vi "Lock_LO_RevB_digitalPLL_NAOJ_2.vi"(0 "ObjHandle in":u32, 2 "LO_FREQ_SET":T1={"YTO Low freq. [GHz]"=12.17, "YTO High freq. [GHz]"=14.833, "Kvco"=1, "Lock Pol."=0, "SET LO FREQ"=25.0, "Multiplier"=3.0, "YTO coarse tune(HEX)"=0, "YTO coarse( FREQ)"=25.0, "NULL PLL INTEGRATOR"=FALSE} {"YTO coarse( FREQ)" min=25 max=150 step=0.0001 format="%.3f"; "YTO coarse tune(HEX)" format="%x"; "Multiplier" min=3 max=6 step=3; "SET LO FREQ" min=25 max=150 step=0.0001 format="%.3f"; "Lock Pol." items=["Lower", "Upper"]; "Kvco" items=["7.5MHz/V", "15MHz/V"]; "YTO High freq. [GHz]" format="%.3f"; "YTO Low freq. [GHz]" format="%.3f"}, 5 "error in (no error)":errorcluster, 10 "Slave Node in":cluster{"Address":i16, "Serial Number":i8[]}={"Address"=19, "Serial Number"=[16, 71, 55, 76, 1, 8, 0, -15]} {"Serial Number" format="%.0x"; "Address" format="%.0x"}, 12 "Cartridge band":u32 max=10 step=1) -> (15 "LO_FREQ_output":T1={"YTO Low freq. [GHz]"=12.17, "YTO High freq. [GHz]"=14.833, "Kvco"=1, "Lock Pol."=0, "SET LO FREQ"=25.0, "Multiplier"=3.0, "YTO coarse tune(HEX)"=0, "YTO coarse( FREQ)"=25.0, "NULL PLL INTEGRATOR"=FALSE} {"YTO coarse( FREQ)" min=25 max=150 step=0.0001 format="%.3f"; "YTO coarse tune(HEX)" format="%x"; "Multiplier" min=3 max=6 step=3; "SET LO FREQ" min=25 max=150 step=0.0001 format="%.3f"; "Lock Pol." items=["Lower", "Upper"]; "Kvco" items=["7.5MHz/V", "15MHz/V"]; "YTO High freq. [GHz]" format="%.3f"; "YTO Low freq. [GHz]" format="%.3f"}, 16 "YTO final Freq [GHz]":sgl format="%.4f", 17 "YTO fine  Freq [GHz]":sgl format="%.4f", 19 "error out":errorcluster)   [LabVIEW 2017]
panel:
  in  "step(GHz)":sgl=0.001
  out "l":dbl
  out "ObjHandle out":u32
  # "LO freq. [GHz]"
  # "ZERO Intgrtr"
  # "LO freq. [GHz]"
  # "ZERO Intgrtr"
  # "Node Address"
  # "Serial Number"
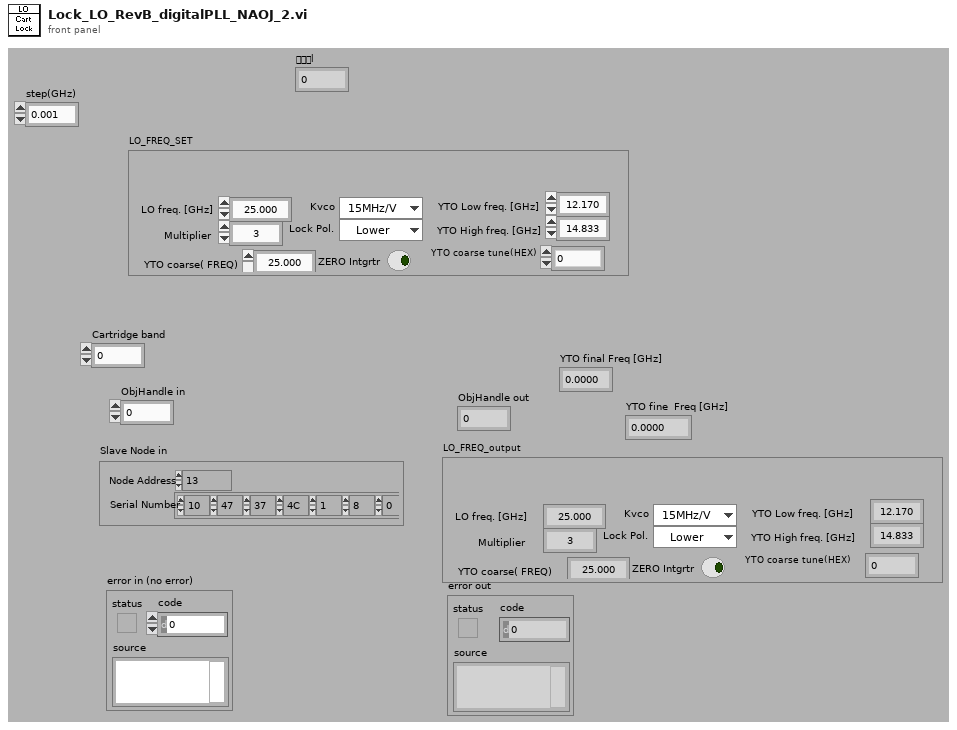
[diagram p1: front panel]
types:
  T1 = cluster{"YTO Low freq. [GHz]":sgl, "YTO High freq. [GHz]":sgl, "Kvco":u16, "Lock Pol.":u16, "SET LO FREQ":sgl, "Multiplier":sgl, "YTO coarse tune(HEX)":u16, "YTO coarse( FREQ)":sgl, "NULL PLL INTEGRATOR":bool}
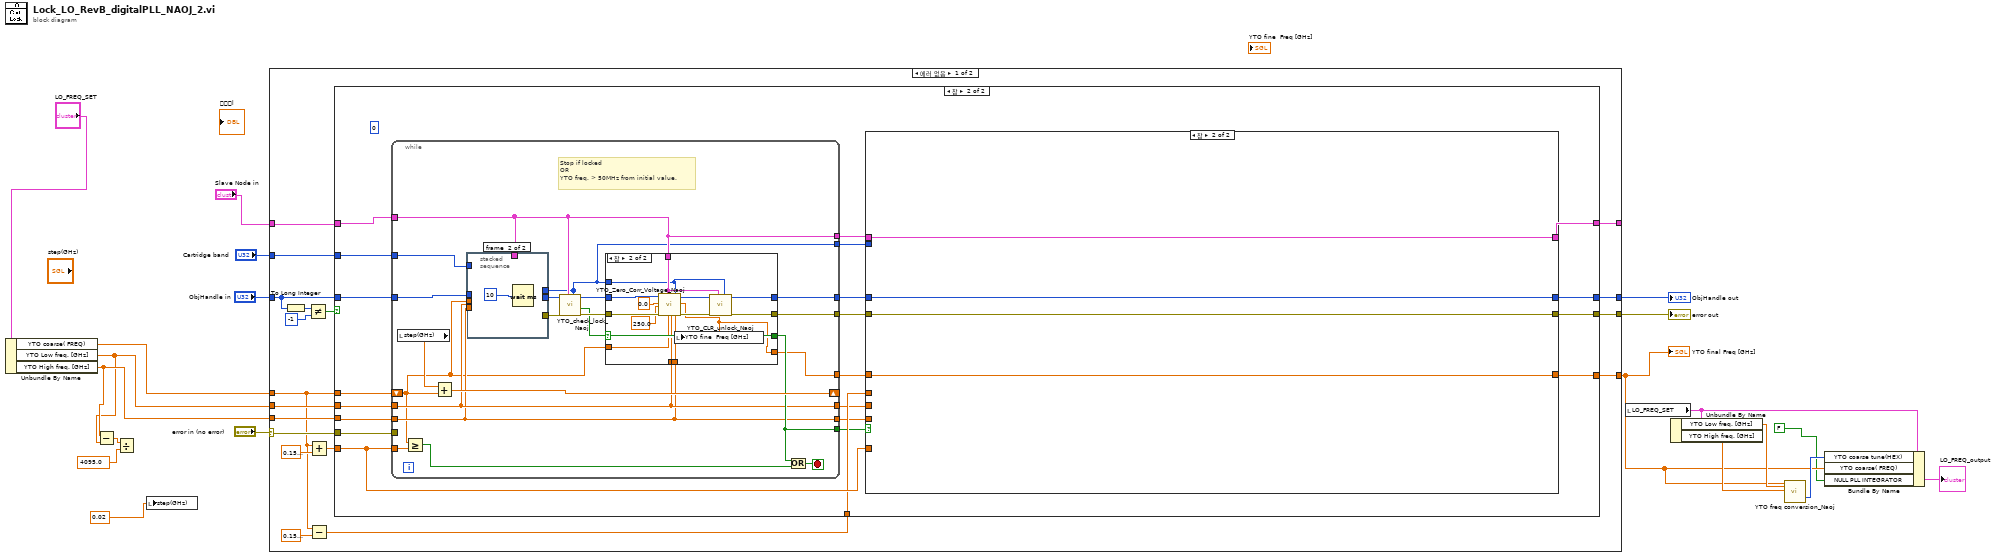
[diagram p0: block diagram]
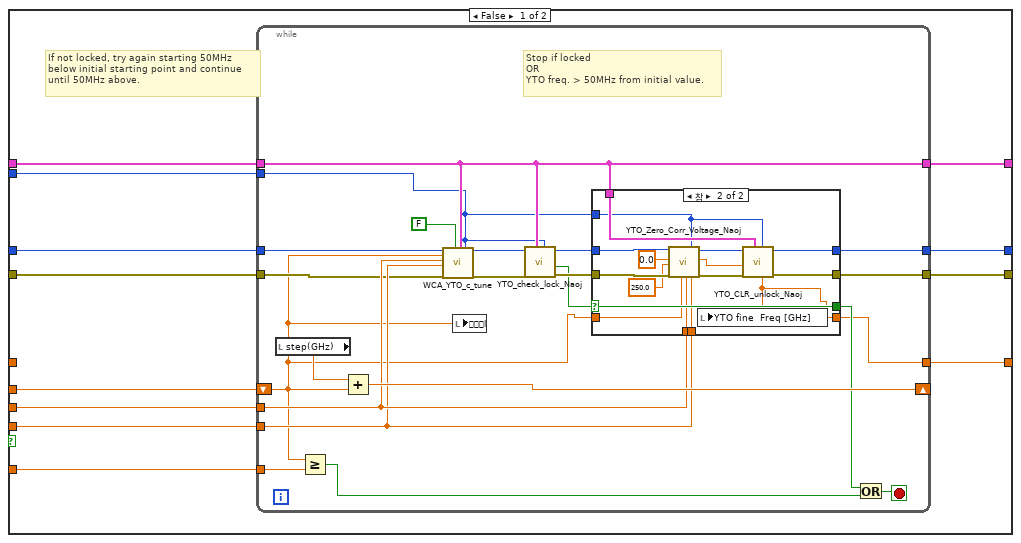
[diagram p3: hidden frame]
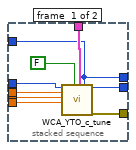
[diagram p5: hidden frame]
diagram:
  n1 = Unbundle By Name("LO_FREQ_SET") -> ("YTO coarse( FREQ)"=w13:sgl, "YTO Low freq. [GHz]"=w2:sgl, "YTO High freq. [GHz]"=w3:sgl)
  n2 = Subtract(x=w3, y=w2) -> (x-y=w5:sgl)
  n3 = Divide(x=w5, y=4095.0) -> ()  [unwired: 1 out]
  n4 = local write "step(GHz)"(0.02) -> ()
  n5 = case shown="에러 없음" "error in (no error)" {
    selector: "error in (no error)" -> [w35 w174]
    tunnel: "ObjHandle in" -> [w34 w172]
    tunnel: "Slave Node in" -> [w33 w173]
    tunnel: w2 -> [w32 _]
    tunnel: w3 -> [w31 _]
    tunnel: w13 -> [w23 _]
    tunnel: [w30 w172] -> w17
    tunnel: [w29 w173] -> _
    tunnel: [w28 w174] -> w18
    tunnel: [w25 sgl -1.0 ("SET YTO COARSE TUNE")] -> w7
    tunnel: "Cartridge band" -> [w21 _]
    frame No Error {
      n6 = To Long Integer(number=w34) -> (32bit integer=w37:i32)
      n7 = Not Equal?(x=w37, y=-1) -> (x != y?=w36:bool)
      n8 = Add(x=w23, y=sgl 0.15) -> (x+y=w26:sgl)
      n9 = Subtract(x=w23, y=sgl 0.15) -> (x-y=w22:sgl)
      n10 = case shown="참" w36 {
        tunnel: w35 -> [w40 w60]
        tunnel: w34 -> [w42 w45]
        tunnel: w33 -> [w41 w46]
        tunnel: w32 -> [_ w62]
        tunnel: w31 -> [_ w61]
        tunnel: w23 -> [_ w63]
        tunnel: [w42 w56] -> w30
        tunnel: [w41 w55] -> w29
        tunnel: [w40 w57] -> w28
        tunnel: w26 -> [_ w59]
        tunnel: [sgl -1.0 ("SET YTO COARSE TUNE") w58] -> w25
        tunnel: w22 -> [_ w54]
        tunnel: w21 -> [_ w44]
        frame False {
        }
        frame True {
          (unwired) 0 ("SET NULL PLL INTEGRATOR")
          n11 = while {
            tunnel: w45 -> [w123]
            tunnel: w62 -> [w129]
            tunnel: w61 -> [w128]
            tunnel: w60 -> [_]
            shift-right: [w135] -> _
            shift-left: w63 -> [w122]
            tunnel: w59 -> [w134]
            tunnel: [w121] -> w50
            tunnel: [w132] -> w51
            tunnel: [w131] -> w52
            tunnel: [w127] -> w53
            tunnel: [w130] -> w49
            tunnel: [w129] -> w48
            tunnel: [w128] -> w47
            tunnel: w46 -> [w127]
            tunnel: w44 -> [w125]
            tunnel: [w124] -> w43
            stop <- w136 stop-if-true
            # "Stop if locked\nOR\nYTO freq. > 50MHz from initial value."
            n12 = local read "step(GHz)"() -> (w126:sgl)
            n13 = Greater Or Equal?(x=w122, y=w134) -> (x >= y?=w133:bool)
            n14 = Add(x=w126, y=w122) -> (x+y=w135:sgl)
            n15 = stacked-sequence {
              tunnel: [w142 _] -> w141
              tunnel: [w150 _] -> w140
              tunnel: w129 -> [w148 _]
              tunnel: w128 -> [w147 _]
              tunnel: w122 -> [w146 _]
              tunnel: w127 -> [w145 _]
              tunnel: w125 -> [w144 _]
              tunnel: [w144 _] -> w124
              tunnel: w123 -> [w143 _]
              frame #0 {
                n16 = call "WCA_YTO_c_tune.vi"("ObjHandle in"=w143, "SET YTO COARSE TUNE"=w146, "YTO Low freq. [GHz]"=w148, "YTO High freq. [GHz]"=w147, "LO locked?"=FALSE, "Slave Node in"=w145, "Cartridge band"=w144) -> ("ObjHandle out"=w142:u32, "error out"=w150:errorcluster)  [unwired: 11 in]
              }
              frame #1 {
                n17 = Wait (ms)(milliseconds to wait=10) -> ()  [unwired: 1 out]
              }
            }
            n18 = call "YTO_check_lock_Naoj.vi"("Cartridge band"=w124, "Slave Node in"=w127, "error IO"=w140, "ObjHandle in"=w141) -> ("error"=w138:errorcluster, "Lock"=w137:bool, "ObjHandle out"=w139:u32)  [unwired: 5 in]
            n19 = case shown="참" w137 {
              selector: w137 -> [w155 w166]
              tunnel: w139 -> [w154 w170]
              tunnel: w138 -> [w153 w169]
              tunnel: [w155 w166] -> w130
              tunnel: [w154 w161] -> w131
              tunnel: [w153 w160] -> w132
              tunnel: w129 -> [_ w165]
              tunnel: w128 -> [_ w164]
              tunnel: w127 -> [_ w159]
              tunnel: w124 -> [_ w158]
              tunnel: [w152 w156] -> w121
              tunnel: w122 -> [w152 w157]
              frame False {
              }
              frame True {
                n20 = call "YTO_Zero_Corr_Voltage_Naoj.vi"("ObjHandle in"=w170, "Desired YTO Corr Volt [V]"=0.0, "Voltage Limit [mV]"=250.0, "error in (no error)"=w169, "Slave Node in"=w159, "SET YTO COARSE TUNE"=w157, "YTO Low freq. [GHz]"=w165, "Cartridge band"=w158, "YTO High freq. [GHz]"=w164) -> ("ObjHandle out"=w162:u32, "YTO_fine"=w156:dbl, "error out"=w163:errorcluster)  [unwired: 7 in, 1 out]
                n21 = local write "YTO fine  Freq [GHz]"(w156) -> ()
                n22 = call "YTO_CLR_unlock_Naoj.vi"("Cartridge band"=w158, "Slave Node in"=w159, "error IO"=w163, "ObjHandle in"=w162) -> ("error"=w160:errorcluster, "ObjHandle out"=w161:u32)  [unwired: 6 in]
              }
            }
            n23 = Or(x=w130, y=w133) -> (x .or. y?=w136:bool)
          }
          n24 = case shown="참" w49 {
            tunnel: w53 -> [w75 w120]
            tunnel: [w68 w120] -> w55
            tunnel: w52 -> [w74 w119]
            tunnel: [w67 w119] -> w56
            tunnel: w51 -> [w73 w118]
            tunnel: [w66 w118] -> w57
            tunnel: w50 -> [_ w117]
            tunnel: [w65 w117] -> w58
            tunnel: w48 -> [w72 _]
            tunnel: w47 -> [w71 _]
            tunnel: w59 -> [w70 _]
            tunnel: w54 -> [w69 _]
            tunnel: w43 -> [w64 _]
            frame False {
              # "If not locked, try again starting 50MHz\nbelow initial starting point and continue\nuntil 50MHz above."
              n25 = while {
                tunnel: w74 -> [w97]
                tunnel: w72 -> [w84]
                tunnel: w71 -> [w83]
                tunnel: w75 -> [w80]
                shift-right: [w90] -> _
                shift-left: w69 -> [w77]
                tunnel: w70 -> [w89]
                tunnel: [w76] -> w65
                tunnel: [w86] -> w66
                tunnel: [w85] -> w67
                tunnel: [w80] -> w68
                tunnel: w73 -> [w81]
                tunnel: w64 -> [w78]
                stop <- w91 stop-if-true
                # "Stop if locked\nOR\nYTO freq. > 50MHz from initial value."
                n26 = local read "step(GHz)"() -> (w79:sgl)
                n27 = Greater Or Equal?(x=w77, y=w89) -> (x >= y?=w87:bool)
                n28 = Add(x=w79, y=w77) -> (x+y=w90:sgl)
                n29 = call "WCA_YTO_c_tune.vi"("ObjHandle in"=w97, "SET YTO COARSE TUNE"=w77, "YTO Low freq. [GHz]"=w84, "YTO High freq. [GHz]"=w83, "error in (no error)"=w81, "LO locked?"=FALSE, "Slave Node in"=w80, "Cartridge band"=w78) -> ("ObjHandle out"=w96:u32, "error out"=w95:errorcluster)  [unwired: 10 in]
                n30 = local write "l"(w77) -> ()
                n31 = call "YTO_check_lock_Naoj.vi"("Cartridge band"=w78, "Slave Node in"=w80, "error IO"=w95, "ObjHandle in"=w96) -> ("error"=w93:errorcluster, "Lock"=w92:bool, "ObjHandle out"=w94:u32)  [unwired: 5 in]
                n32 = case shown="참" w92 {
                  selector: w92 -> [w101 w112]
                  tunnel: w94 -> [w100 w116]
                  tunnel: w93 -> [w99 w115]
                  tunnel: w80 -> [_ w105]
                  tunnel: [w101 w112] -> w88
                  tunnel: [w100 w107] -> w85
                  tunnel: [w99 w106] -> w86
                  tunnel: w84 -> [_ w111]
                  tunnel: w83 -> [_ w110]
                  tunnel: w78 -> [_ w104]
                  tunnel: [w98 w102] -> w76
                  tunnel: w77 -> [w98 w103]
                  frame False {
                  }
                  frame True {
                    n33 = call "YTO_Zero_Corr_Voltage_Naoj.vi"("ObjHandle in"=w116, "Desired YTO Corr Volt [V]"=0.0, "Voltage Limit [mV]"=250.0, "error in (no error)"=w115, "SET YTO COARSE TUNE"=w103, "YTO Low freq. [GHz]"=w111, "Cartridge band"=w104, "YTO High freq. [GHz]"=w110) -> ("ObjHandle out"=w108:u32, "YTO_fine"=w102:dbl, "error out"=w109:errorcluster)  [unwired: 8 in, 1 out]
                    n34 = local write "YTO fine  Freq [GHz]"(w102) -> ()
                    n35 = call "YTO_CLR_unlock_Naoj.vi"("Cartridge band"=w104, "Slave Node in"=w105, "error IO"=w109, "ObjHandle in"=w108) -> ("error"=w106:errorcluster, "ObjHandle out"=w107:u32)  [unwired: 6 in]
                  }
                }
                n36 = Or(x=w88, y=w87) -> (x .or. y?=w91:bool)
              }
            }
            frame True {
            }
          }
        }
      }
    }
    frame Error {
    }
  }
  "error out" <- w18
  "ObjHandle out" <- w17
  "YTO final Freq [GHz]" <- w7
  n37 = local read "LO_FREQ_SET"() -> (w9:T1)
  n38 = Unbundle By Name(w9) -> ("YTO Low freq. [GHz]"=w12:sgl, "YTO High freq. [GHz]"=w11:sgl)
  n39 = call "YTO freq conversion_Naoj.vi"("YTO desired frequency"=w7, "YTO freq Min"=w12, "YTO freq. Max"=w11) -> ("YTO Coarse tune"=w10:u16)  [unwired: 16 in]
  n40 = Bundle By Name(cluster=w9, "YTO coarse tune(HEX)"=w10, "YTO coarse( FREQ)"=w7, "NULL PLL INTEGRATOR"=FALSE) -> (→"LO_FREQ_output":T1)
